vi "Configure Bandwidth.vi"(0 "VISA resource name":refnum<visa-resource-name>, 1 "CISPR Resolution Bandwidth (9000:9kHz)":dbl(ring)=9000.0 items=["200"=200.0, "9K"=9000.0, "120K"=120000.0, "1M"=1000000.0], 2 "Resolution Bandwidth Mode (0:Normal)":i32(ring) items=["Normal", "CISPR"], 3 "Enable Resolution Bandwidth  (F:Disable)":bool, 5 "Auto Resolution Bandwidth  (T:Enable)":bool=TRUE, 7 "Resolution Bandwidth (300:300Hz)":dbl(ring)=10000.0 items=["1"=1.0, "3"=3.0, "10"=10.0, "30"=30.0, "100"=100.0, "300"=300.0, "1K"=1000.0, "3K"=3000.0, "10K"=10000.0, "30K"=30000.0, "100K"=100000.0, "300K"=300000.0, "1M"=1000000.0, "3M"=3000000.0, "50K"=50000.0, "5M"=5000000.0, "10M"=10000000.0, "20M"=20000000.0, "31.25M"=31250000.0], 9 "Auto Video Bandwidth (0:Auto)":i32(ring) items=["Auto", "Set Bandwidth", "Off"], 11 "error in (no error)":errorcluster, 12 "Video Bandwidth (30000:30KHz)":dbl(ring)=10000.0 items=["1"=1.0, "3"=3.0, "10"=10.0, "30"=30.0, "100"=100.0, "300"=300.0, "1K"=1000.0, "3K"=3000.0, "10K"=10000.0, "30K"=30000.0, "100K"=100000.0, "300K"=300000.0, "1M"=1000000.0, "3M"=3000000.0, "10M"=10000000.0, "5K"=5000.0], 13 "Video Bandwidth Mode (0:Video)":i32(ring) items=["Video", "Power"]) -> (4 "VISA resource name out":refnum<visa-resource-name>, 15 "error out":errorcluster)   [LabVIEW 2023, in "Anritsu Signal Analyzer Series.lvlib"]
doc: "Configures the bandwidth settings of the spectrum analyzer."
uses:
  Anritsu Signal Analyzer Series.lvlib
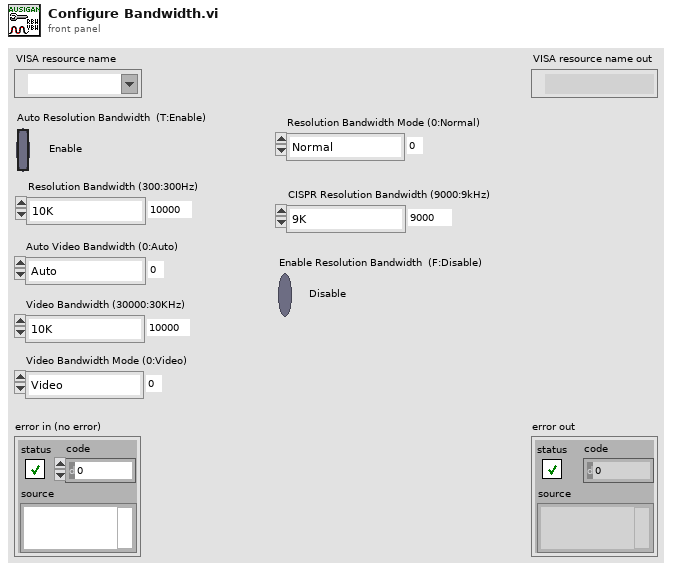
[diagram p1: front panel]
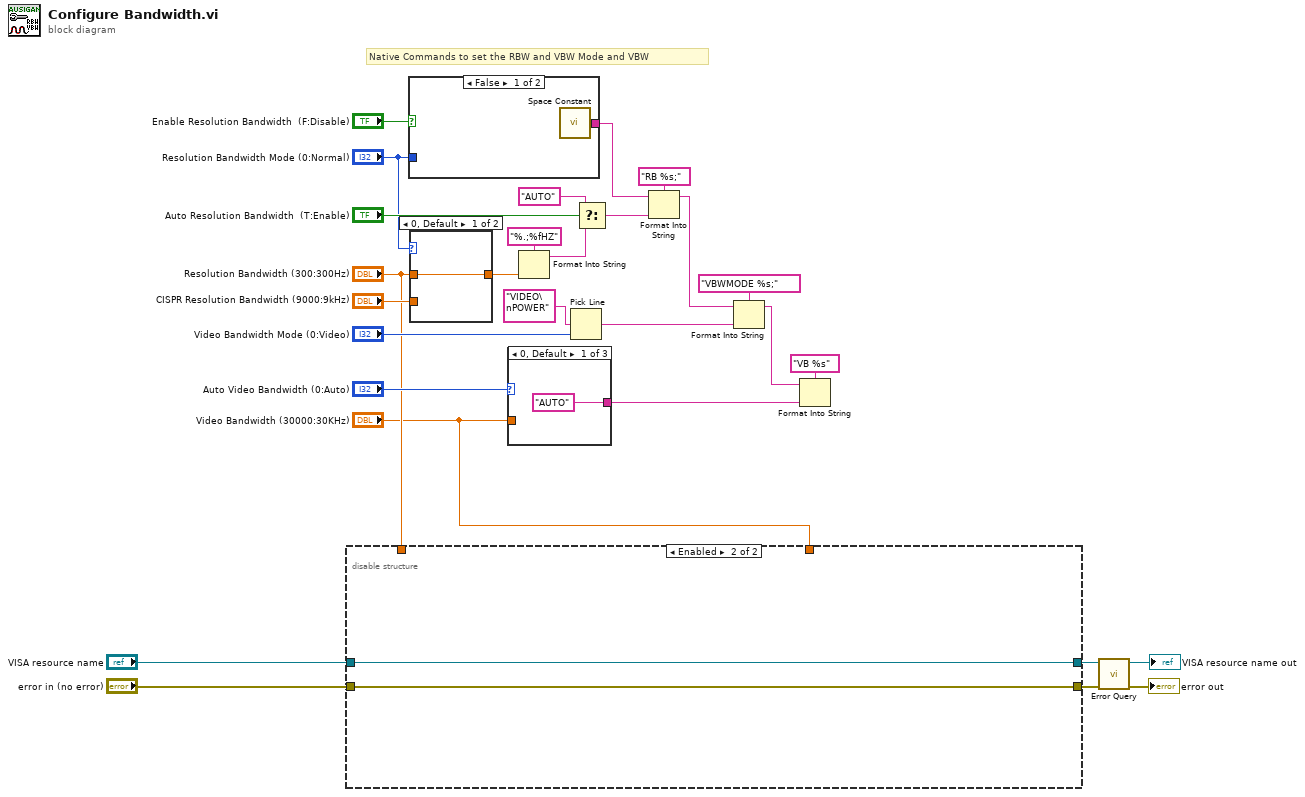
[diagram p0: block diagram]
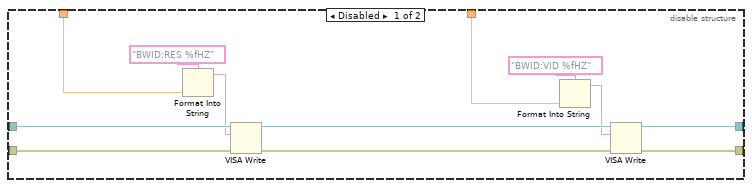
[diagram p2: hidden frame]
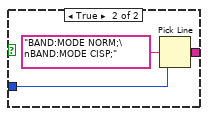
[diagram p3: hidden frame]
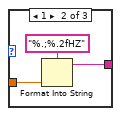
[diagram p5: hidden frame]
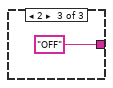
[diagram p6: hidden frame]
diagram:
  # "Native Commands to set the RBW and VBW Mode and VBW"
  n1 = disable-structure shown="Enabled" {
    disable-tunnel: "VISA resource name" -> [w40 w42]
    disable-tunnel: "error in (no error)" -> [w39 w41]
    disable-tunnel: [w36 w41] -> w4
    disable-tunnel: [w34 w42] -> w3
    disable-tunnel: "Resolution Bandwidth (300:300Hz)" -> [w32 _]
    disable-tunnel: "Video Bandwidth (30000:30KHz)" -> [w29 _]
    frame Disabled {
      n2 = Format Into String(format string="BWID:RES %fHZ" ("Format String"), w32) -> (resulting string=w33:string)  [unwired: 2 in, 1 out]
      n3 = VISA Write(VISA resource name=w40, write buffer=w33, error in (no error)=w39) -> (VISA resource name out=w35:refnum<visa-resource-name>, error out=w37:errorcluster)  [unwired: 1 out]
      n4 = Format Into String(format string="BWID:VID %fHZ" ("Format String"), w29) -> (resulting string=w30:string)  [unwired: 2 in, 1 out]
      n5 = VISA Write(VISA resource name=w35, write buffer=w30, error in (no error)=w37) -> (VISA resource name out=w34:refnum<visa-resource-name>, error out=w36:errorcluster)  [unwired: 1 out]
    }
    frame Enabled {
    }
  }
  n6 = case shown="False" "Enable Resolution Bandwidth  (F:Disable)" {
    tunnel: [w43 w45] -> w9
    tunnel: "Resolution Bandwidth Mode (0:Normal)" -> [_ w44]
    frame False {
      n7 = call <vilib>:"Space Constant.vi"() -> ("String"=w43:string)
    }
    frame True {
      n8 = Pick Line(multi-line string="BAND:MODE NORM;\nBAND:MODE CISP;", line index=w44) -> (output string=w45:string)  [unwired: 1 in]
    }
  }
  n9 = case shown="0, Default" "Resolution Bandwidth Mode (0:Normal)" {
    tunnel: "Resolution Bandwidth (300:300Hz)" -> [w47 _]
    tunnel: [w47 w48] -> w7
    tunnel: "CISPR Resolution Bandwidth (9000:9kHz)" -> [_ w48]
    frame 0, Default {
    }
    frame 1 {
    }
  }
  n10 = case shown="0, Default" "Auto Video Bandwidth (0:Auto)" {
    tunnel: ["AUTO" w51 "OFF"] -> w20
    tunnel: "Video Bandwidth (30000:30KHz)" -> [_ w50 _]
    frame 0, Default {
    }
    frame 1 {
      n11 = Format Into String(format string="%.;%.2fHZ" ("Format String"), w50) -> (resulting string=w51:string)  [unwired: 2 in, 1 out]
    }
    frame 2 {
    }
  }
  n12 = Format Into String(format string="%.;%fHZ" ("Format String"), w7) -> (resulting string=w14:string)  [unwired: 2 in, 1 out]
  n13 = Pick Line(multi-line string="VIDEO\nPOWER" ("_Case0"), line index="Video Bandwidth Mode (0:Video)") -> (output string=w11:string)  [unwired: 1 in]
  n14 = Select(t="AUTO", s="Auto Resolution Bandwidth  (T:Enable)", f=w14) -> (s? t:f=w13:string)
  n15 = Format Into String(format string="RB %s;" ("_CommandSet"), initial string=w9, w13) -> (resulting string=w21:string)  [unwired: 1 in, 1 out]
  n16 = Format Into String(format string="VBWMODE %s;" ("_CommandSet"), initial string=w21, w11) -> (resulting string=w19:string)  [unwired: 1 in, 1 out]
  n17 = Format Into String(format string="VB %s" ("_CommandSet"), initial string=w19, w20) -> ()  [unwired: 1 in, 2 out]
  n18 = call "Error Query.vi"("error in (no error)"=w4, "VISA resource name"=w3) -> ("error out"=→"error out":errorcluster, "VISA resource name out"=→"VISA resource name out":refnum<visa-resource-name>)  [unwired: 6 in, 2 out]
